vi "ValueRGBIntoSting(SubVI).vi"(1 "B":string, 2 "G":string, 3 "R":string) -> (0 "RGB String":string)   [LabVIEW 2018]
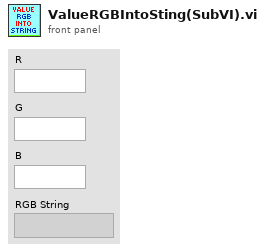
[diagram p1: front panel]
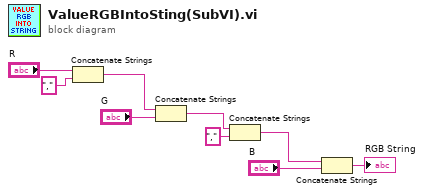
[diagram p0: block diagram]
diagram:
  n1 = Concatenate Strings("R", "," ("string")) -> (w6:string)
  n2 = Concatenate Strings(w6, "G") -> (w5:string)
  n3 = Concatenate Strings(w5, "," ("string")) -> (w3:string)
  n4 = Concatenate Strings(w3, "B") -> (→"RGB String":string)
